vi "Point&Path@SetPathIO__Parameter.vi"(1 "ParamterIn":string) -> (0 "ParamterOut":string)   [LabVIEW 2020]
panel:
  in  "Index":string(combo)
  in  "Type":string(combo)
  in  "Parameter":string(combo)
  in  "PointName":string(combo)
  in  "Confirm":bool
  # "Point&Path@SetPathIO $Point[$Index], On $IO\nPoint&Path@SetPathIO $Point[$Index], Off $IO\nPoint&Path@SetPathIO $Point[$Index], Delay $second\n$IO is 0~3, and $Delay is from 0.001~60"
  # "["
  # "]"
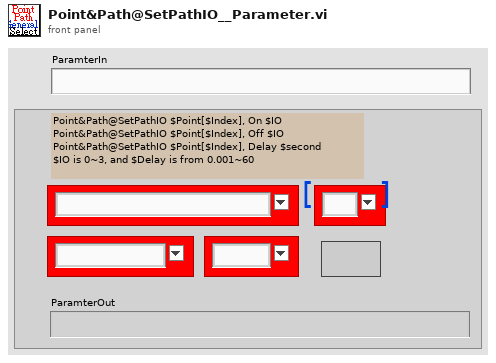
[diagram p1: front panel]
types:
  T1 = enum16{"Get", "UpdatePointS", "Init", "UpdateIndex", "GetCurrent&Index+1", "GetWithIndex", "ChkLast", "GetCurrent"}
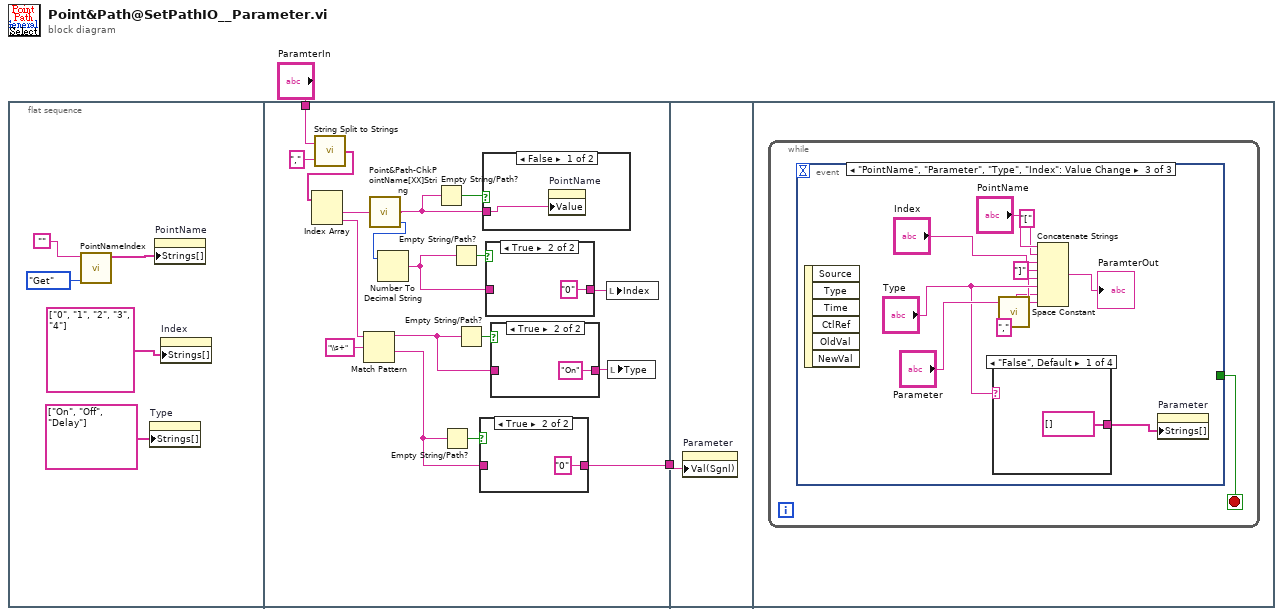
[diagram p0: block diagram]
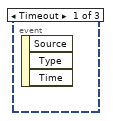
[diagram p6: hidden frame]
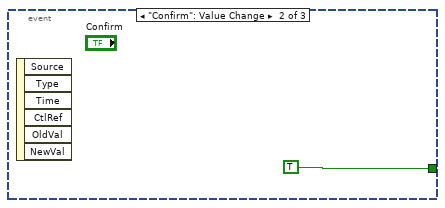
[diagram p7: hidden frame]
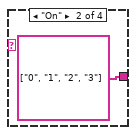
[diagram p8: hidden frame]
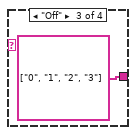
[diagram p9: hidden frame]
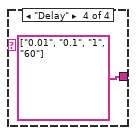
[diagram p10: hidden frame]
diagram:
  n1 = flat-sequence {
    tunnel: "ParamterIn" -> [w20]
    tunnel: [w23] -> w1
    tunnel: w1 -> [w33]
    frame #0 {
      n2 = call "PointNameIndex.vi"("OP"=T1."Get", "PointName"="") -> ("PointNameList"=w4:string[])  [unwired: 4 in, 5 out]
      n3 = property on="Type" class="CmbBox"("Strings[]"=string[] ["On", "Off", "Delay"] ("Strings []")) -> ()  [unwired: 2 in, 2 out]
      n4 = property on="PointName" class="CmbBox"("Strings[]"=w4) -> ()  [unwired: 2 in, 2 out]
      n5 = property on="Index" class="CmbBox"("Strings[]"=string[] ["0", "1", "2", "3", "4"] ("Strings []")) -> ()  [unwired: 2 in, 2 out]
    }
    frame #1 {
      n6 = call "String Split to Strings.vi"("search string/char (-)"=",", "String"=w20) -> ("Array"=w18:string[])
      n7 = Index Array(array=w18) -> (element #1=w11:string, element #2=w12:string)  [unwired: 2 in]
      n8 = Match Pattern(string=w12, regular expression="\\s+") -> (before substring=w14:string, after substring=w13:string)  [unwired: 1 in, 2 out]
      n9 = call "Point&Path-ChkPointName[XX]String.vi"("PointName[XX]"=w11) -> ("Index"=w9:i32, "PointName"=w10:string)  [unwired: 1 in, 2 out]
      n10 = Number To Decimal String(number=w9) -> (decimal integer string=w8:string)  [unwired: 1 in]
      n11 = Empty String/Path?(string/path=w10) -> (empty?=w25:bool)
      n12 = Empty String/Path?(string/path=w13) -> (empty?=w24:bool)
      n13 = Empty String/Path?(string/path=w8) -> (empty?=w17:bool)
      n14 = Empty String/Path?(string/path=w14) -> (empty?=w22:bool)
      n15 = case shown="True" w24 {
        tunnel: [w30 "0"] -> w23
        tunnel: w13 -> [w30 _]
        frame False {
        }
        frame True {
        }
      }
      n16 = case shown="False" w25 {
        tunnel: w10 -> [w32 _]
        frame False {
          n17 = property on="PointName" class="CmbBox"("Value"=w32) -> ()  [unwired: 2 in, 2 out]
        }
        frame True {
        }
      }
      n18 = case shown="True" w17 {
        tunnel: [w26 "0" ("ParamterIn")] -> w16
        tunnel: w8 -> [w26 _]
        frame False {
        }
        frame True {
        }
      }
      n19 = case shown="True" w22 {
        tunnel: [w28 "On" ("ParamterIn")] -> w21
        tunnel: w14 -> [w28 _]
        frame False {
        }
        frame True {
        }
      }
      n20 = local write "Index"(w16) -> ()
      n21 = local write "Type"(w21) -> ()
    }
    frame #2 {
      n22 = property on="Parameter" class="CmbBox"("Val(Sgnl)"=w33) -> ()  [unwired: 2 in, 2 out]
    }
    frame #3 {
      n23 = while {
        stop <- w34 stop-if-true
        n24 = event shown="[2] \"PointName\", \"Parameter\", \"Type\", \"Index\": Value Change" {
          selector: _ -> [_ _ _]
          dyn-events: _ -> [_ _ _]
          timeout: _ -> [_ _ _]
          tunnel: [_ TRUE _] -> w34
          event Timeout {
            n25 = event-data() -> ()  [unwired: 1 in, 3 out]
          }
          event "Confirm": Value Change {
            n26 = event-data() -> ()  [unwired: 1 in, 6 out]
          }
          event "PointName", "Parameter", "Type", "Index": Value Change {
            n27 = event-data() -> ()  [unwired: 1 in, 6 out]
            n28 = case shown="\"False\", Default" "Type" {
              tunnel: [string[] [] ("Strings []") string[] ["0", "1", "2", "3"] ("Strings []") string[] ["0", "1", "2", "3"] ("Strings []") string[] ["0.01", "0.1", "1", "60"] ("Strings []")] -> w42
              frame "False", Default {
              }
              frame "On" {
              }
              frame "Off" {
              }
              frame "Delay" {
              }
            }
            n29 = call <vilib>:"Space Constant.vi"() -> ("String"=w38:string)
            n30 = Concatenate Strings("PointName", "[" ("string"), "Index", "]" ("string"), "," ("string"), "Type", w38, "Parameter") -> (→"ParamterOut":string)
            n31 = property on="Parameter" class="CmbBox"("Strings[]"=w42) -> ()  [unwired: 2 in, 2 out]
          }
        }
      }
    }
  }
